vi "Simple AAV.vi"() -> ()   [LabVIEW 2012]
doc: "This VI acquires, analyzes, and presents data. It is a solution VI to an exercise in the LabVIEW Core I course. Refer to the course manual for instructions."
uses:
  Instance           2 18Saved   Simple AAP .vi
  Instance           3 18Saved   Simple AAP .vi
panel:
  out "Waveform Graph":dynamicdata(graph)
  out "Average Value":dbl
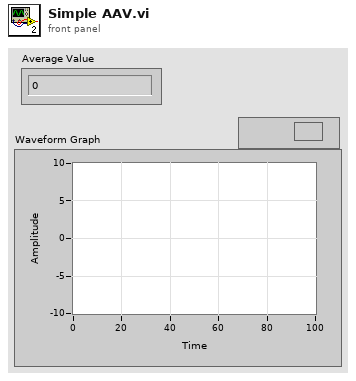
[diagram p1: front panel]
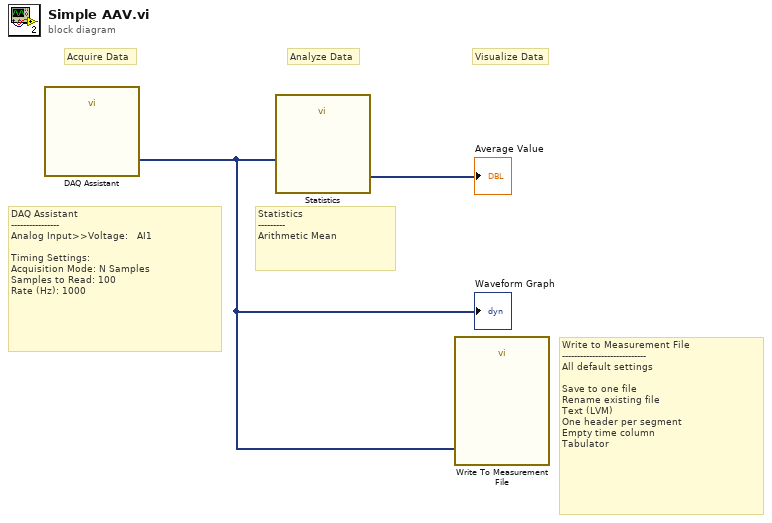
[diagram p0: block diagram]
diagram:
  # "Statistics\n---------\nArithmetic Mean"
  # "Write to Measurement File\n----------------------------\nAll default settings\n\nSave to one file\nRename existing file\nText (LVM)\nOne header per segment\nEmpty time column\nTabulator"
  # "DAQ Assistant\n----------------\nAnalog Input>>Voltage:   AI1\n\nTiming Settings:\nAcquisition Mode: N Samples\nSamples to Read: 100\nRate (Hz): 1000"
  # "Visualize Data"
  # "Analyze Data"
  # "Acquire Data"
  n1 = call "DAQ Assistant"() -> ("data"=w2:dynamicdata)  [unwired: 9 in, 2 out]
  "Waveform Graph" <- w2
  n2 = call "Statistics"("Signals"=w2) -> ("Arithmetic Mean"=→"Average Value":dynamicdata)  [unwired: 25 in, 1 out]
  n3 = call "Write To Measurement File"("Signals"=w2) -> ()  [unwired: 8 in, 3 out]
